vi "DK240 Goto.vi"(4 "StopRef":refnum<vi>, 5 "error in":errorcluster, 6 "Wavelenght":dbl caption="Longueur \nd'onde (nm)" min=0.0 max=16777000.0 step=0.1 format="%#.2f", 7 "MovingRef":refnum<vi>, 8 "Port":refnum<visa-resource-name>="SPECTRO") -> (0 "error out":errorcluster, 2 "Moving":bool caption="Déplacement\nen cours", 3 "Status":u8)   [LabVIEW 2019]
doc: "Goto - Ce Vi commande au réseaux du monochromateur de pivoter à la longueur d'onde désirée, en nm."
uses:
  <vilib>/Utility/error.llb/DialogType.ctl
  <userlib>/GenProg/WritebyWeakRefBool.vi
  <userlib>/GenProg/ReadbyWeakRefBool.vi
panel:
  in  "StopOp":bool
  out "Cancel":u8
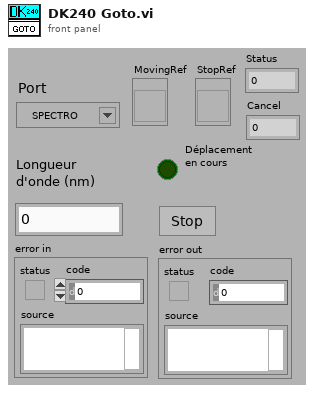
[diagram p1: front panel]
types:
  T1 = enum16{"Commande", "AttendPrêt", "Paramètre", "AttendFin", "Statut", "Fin"}
  T2 = typedef "DialogType.ctl" = u16
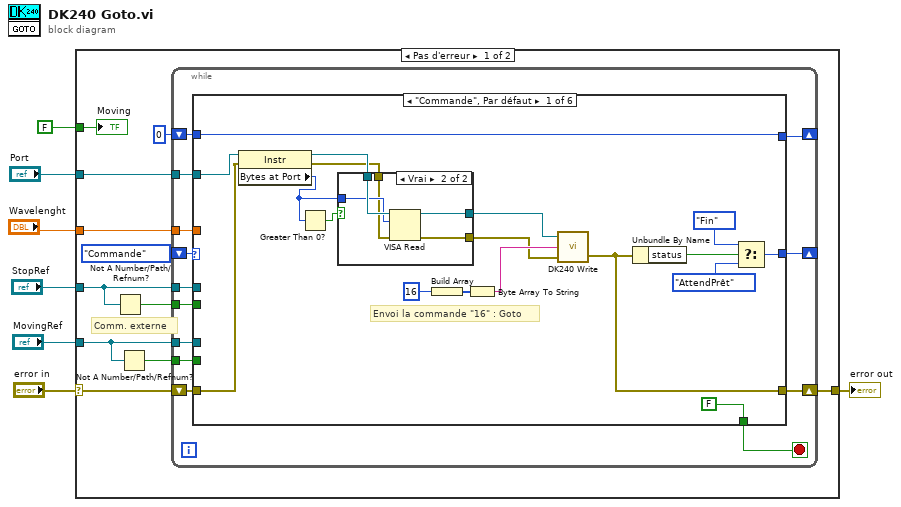
[diagram p0: block diagram]
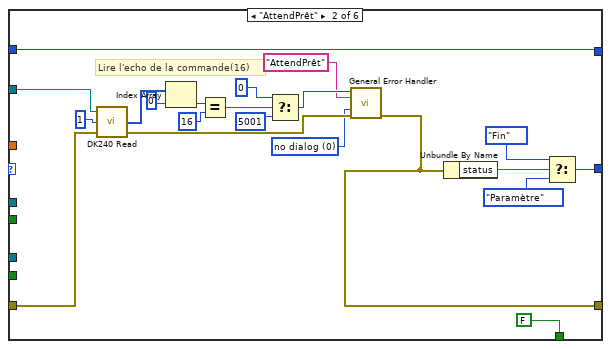
[diagram p3: hidden frame]
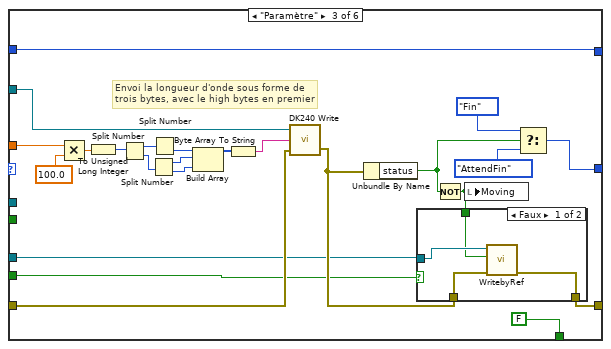
[diagram p4: hidden frame]
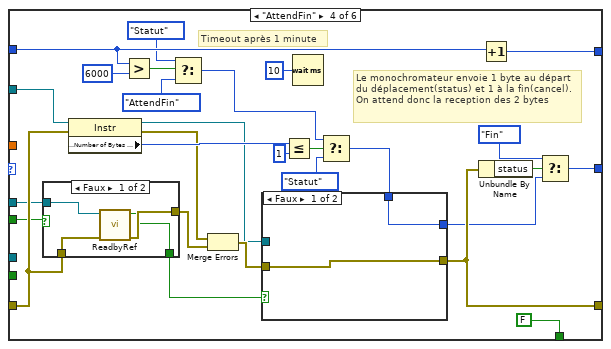
[diagram p6: hidden frame]
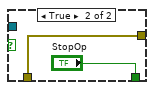
[diagram p7: hidden frame]
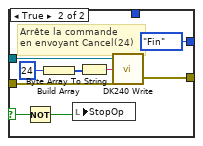
[diagram p8: hidden frame]
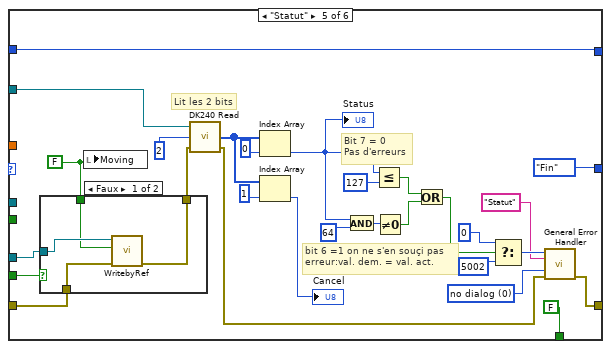
[diagram p9: hidden frame]
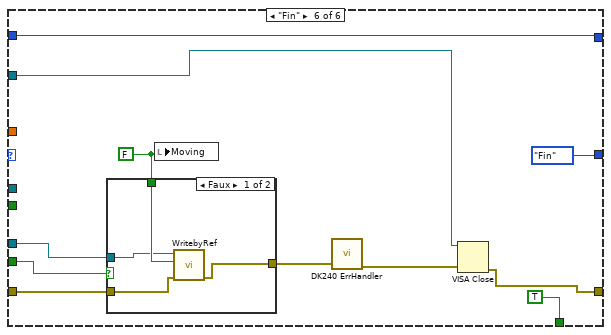
[diagram p11: hidden frame]
diagram:
  n1 = case shown="Pas d'erreur" "error in" {
    selector: "error in" -> [w14 w201]
    tunnel: "Port" -> [w17 _]
    tunnel: "Wavelenght" -> [w16 _]
    tunnel: [w15 w201] -> w6
    tunnel: FALSE ("Moving") -> [w13 _]
    tunnel: "MovingRef" -> [w12 _]
    tunnel: "StopRef" -> [w9 _]
    frame No Error {
      # "Comm. externe"
      n2 = Not A Number/Path/Refnum?(number/path/refnum=w9) -> (NaN/Path/Refnum?=w8:bool)
      n3 = Not A Number/Path/Refnum?(number/path/refnum=w12) -> (NaN/Path/Refnum?=w11:bool)
      n4 = while {
        shift-right: [w27] -> _
        shift-left: T1."Commande" -> [w31]
        tunnel: w17 -> [w30]
        shift-right: [w28] -> w15
        shift-left: w14 -> [w29]
        tunnel: w16 -> [w26]
        tunnel: w12 -> [w24]
        tunnel: w11 -> [w23]
        shift-right: [w22] -> _
        shift-left: 0 -> [w21]
        tunnel: w9 -> [w20]
        tunnel: w8 -> [w19]
        stop <- w25 stop-if-true
        n5 = case shown="\"Commande\", Par défaut" w31 {
          tunnel: w30 -> [w39 w70 w91 w109 w175 w191]
          tunnel: w29 -> [w35 w69 w89 w123 w157 w193]
          tunnel: [w46 w65 w83 w127 w164 w192] -> w28
          tunnel: [w42 w74 w86 w128 T1."Fin" T1."Fin"] -> w27
          tunnel: w26 -> [_ _ w90 _ _ _]
          tunnel: [FALSE FALSE FALSE FALSE FALSE TRUE] -> w25
          tunnel: w24 -> [_ _ w82 _ w154 w190]
          tunnel: w23 -> [_ _ w81 _ w155 w189]
          tunnel: [w40 w57 w78 w118 w152 w187] -> w22
          tunnel: w21 -> [w40 w57 w78 w116 w152 w187]
          tunnel: w20 -> [_ _ _ w110 _ _]
          tunnel: w19 -> [_ _ _ w107 _ _]
          frame "Commande", Default {
            # "Envoi la commande \"16\" : Goto"
            n6 = property class="Instr"(reference=w39, error in=w35) -> (reference out=w37:refnum<visa-resource-name>, error out=w34:errorcluster, "Bytes at Port"=w36:u32)
            n7 = Greater Than 0?(x=w36) -> (x > 0?=w38:bool)
            n8 = case shown="Vrai" w38 {
              tunnel: w37 -> [w50 w56]
              tunnel: w36 -> [_ w55]
              tunnel: w34 -> [w51 w54]
              tunnel: [w51 w53] -> w33
              tunnel: [w50 w52] -> w32
              frame False {
              }
              frame True {
                n9 = VISA Read(VISA resource name=w56, byte count=w55, error in (no error)=w54) -> (VISA resource name out=w52:refnum<visa-resource-name>, error out=w53:errorcluster)  [unwired: 2 out]
              }
            }
            n10 = Build Array(u8 16) -> (w48:u8[])
            n11 = Byte Array To String(unsigned byte array=w48) -> (string=w49:string)
            n12 = call <userlib>:"DK240 Write.vi"("error in"=w33, "String to write"=w49, "Port"=w32) -> ("error out"=w46:errorcluster)  [unwired: 1 in]
            n13 = Unbundle By Name(w46) -> ("status"=w45:bool)
            n14 = Select(t=T1."Fin", s=w45, f=T1."AttendPrêt") -> (s? t:f=w42:T1)
          }
          frame "AttendPrêt" {
            w59 = T2 0 items=["no dialog", "OK message", "continue or stop message", "OK message + warnings", "continue/stop + warnings"] ("type of dialog (OK msg:1)")
            # "Lire l'echo de la commande(16)"
            n15 = call <userlib>:"DK240 Read.vi"("error in"=w69, "Byte count"=u32 1, "Port"=w70) -> ("error out"=w66:errorcluster, "Received Bytes"=w73:u8[])  [unwired: 1 in]
            n16 = Index Array(array=w73, index=0) -> (element=w68:u8)
            n17 = Equal?(x=w68, y=u8 16) -> (x = y?=w64:bool)
            n18 = Select(t=0, s=w64, f=5001 ("t")) -> (s? t:f=w63:i32)
            n19 = call <vilib>:"General Error Handler.vi"("[error code] (0)"=w63, "[error source] (\" \")"="AttendPrêt" ("[error source] (\" \")"), "type of dialog (OK msg:1)"=w59, "error in (no error)"=w66) -> ("error out"=w65:errorcluster)  [unwired: 7 in, 4 out]
            n20 = Unbundle By Name(w65) -> ("status"=w77:bool)
            n21 = Select(t=T1."Fin", s=w77, f=T1."Paramètre") -> (s? t:f=w74:T1)
          }
          frame "Paramètre" {
            # "Envoi la longueur d'onde sous forme de trois bytes, avec le high bytes en premier"
            n22 = Multiply(x=w90, y=100.0) -> (x*y=w99:dbl)
            n23 = To Unsigned Long Integer(number=w99) -> (unsigned 32bit integer=w94:u32)
            n24 = Split Number(x=w94) -> (hi(x)=w93:u16, lo(x)=w92:u16)
            n25 = Split Number(x=w92) -> (hi(x)=w96:u8, lo(x)=w97:u8)
            n26 = Split Number(x=w93) -> (lo(x)=w95:u8)  [unwired: 1 out]
            n27 = Build Array(w95, w96, w97) -> (w100:u8[])
            n28 = Byte Array To String(unsigned byte array=w100) -> (string=w101:string)
            n29 = call <userlib>:"DK240 Write.vi"("error in"=w89, "String to write"=w101, "Port"=w91) -> ("error out"=w84:errorcluster)  [unwired: 1 in]
            n30 = Unbundle By Name(w84) -> ("status"=w79:bool)
            n31 = Not(x=w79) -> (.not. x?=w80:bool)
            n32 = case shown="Faux" w81 {
              tunnel: w82 -> [w105 _]
              tunnel: w84 -> [w103 w106]
              tunnel: [w102 w106] -> w83
              tunnel: w80 -> [w104 _]
              frame False {
                n33 = call-poly <userlib>:"WritebyRef.vi"("error in"=w103, "Valeur"=w104, "Control Ref"=w105) -> ("error out"=w102:errorcluster)  [unwired: 8 in]
              }
              frame True {
              }
            }
            n34 = local write "Moving"(w80) -> ()
            n35 = Select(t=T1."Fin", s=w79, f=T1."AttendFin") -> (s? t:f=w86:T1)
          }
          frame "AttendFin" {
            # "Timeout après 1 minute"
            # "Le monochromateur envoie 1 byte au départ du déplacement(status) et 1 à la fin(cancel). On attend donc la reception des 2 bytes"
            n36 = case shown="Faux" w107 {
              tunnel: w123 -> [w138 w140]
              tunnel: [w135 "StopOp"] -> w120
              tunnel: [w137 w140] -> w119
              tunnel: w110 -> [w136 _]
              frame False {
                n37 = call-poly <userlib>:"ReadbyRef.vi"("error in"=w138, "Control Ref"=w136) -> ("error out"=w137:errorcluster, "Valeur"=w135:bool)  [unwired: 8 in]
              }
              frame True {
              }
            }
            n38 = property class="Instr"(reference=w109, error in=w123) -> (reference out=w108:refnum<visa-resource-name>, error out=w122:errorcluster, "Serial Settings:Number of Bytes at Serial Port"=w134:u32)
            n39 = Greater?(x=w116, y=6000) -> (0:w114:bool)
            n40 = Select(t=T1."Statut", s=w114, f=T1."AttendFin") -> (s? t:f=w111:T1)
            n41 = Merge Errors(w122, w119) -> (w121:errorcluster)
            n42 = Less Or Equal?(x=w134, y=u32 1) -> (x <= y?=w130:bool)
            n43 = Wait (ms)(milliseconds to wait=u32 10) -> ()  [unwired: 1 out]
            n44 = Select(t=w111, s=w130, f=T1."Statut") -> (s? t:f=w125:T1)
            n45 = case shown="Faux" w120 {
              selector: w120 -> [_ w144]
              tunnel: w121 -> [w142 w146]
              tunnel: w108 -> [_ w148]
              tunnel: [w142 w147] -> w127
              tunnel: w125 -> [w141 _]
              tunnel: [w141 T1."Fin"] -> w124
              frame False {
              }
              frame True {
                # "Arrête la commande\nen envoyant Cancel(24)"
                n46 = Not(x=w144) -> (.not. x?=w143:bool)
                n47 = Build Array(u8 24) -> (w150:u8[])
                n48 = local write "StopOp"(w143) -> ()
                n49 = Byte Array To String(unsigned byte array=w150) -> (string=w151:string)
                n50 = call <userlib>:"DK240 Write.vi"("error in"=w146, "String to write"=w151, "Port"=w148) -> ("error out"=w147:errorcluster)  [unwired: 1 in]
              }
            }
            n51 = Unbundle By Name(w127) -> ("status"=w132:bool)
            n52 = Increment(x=w116) -> (x+1=w118:i32)
            n53 = Select(t=T1."Fin", s=w132, f=w124) -> (s? t:f=w128:T1)
          }
          frame "Statut" {
            w169 = T2 0 items=["no dialog", "OK message", "continue or stop message", "OK message + warnings", "continue/stop + warnings"] ("type of dialog (OK msg:1)")
            w153 = FALSE
            # "bit 6 =1 on ne s'en souçi pas \nerreur:val. dem. = val. act."
            # "Bit 7 = 0\nPas d'erreurs"
            # "Lit les 2 bits"
            n54 = case shown="Faux" w155 {
              tunnel: w157 -> [w181 w184]
              tunnel: [w180 w184] -> w156
              tunnel: w154 -> [w183 _]
              tunnel: w153 -> [w182 _]
              frame False {
                n55 = call-poly <userlib>:"WritebyRef.vi"("error in"=w181, "Valeur"=w182, "Control Ref"=w183) -> ("error out"=w180:errorcluster)  [unwired: 8 in]
              }
              frame True {
              }
            }
            n56 = local write "Moving"(w153) -> ()
            n57 = call <userlib>:"DK240 Read.vi"("error in"=w156, "Byte count"=u32 2, "Port"=w175) -> ("error out"=w168:errorcluster, "Received Bytes"=w179:u8[])  [unwired: 1 in]
            n58 = Index Array(array=w179, index=0) -> (element=w160:u8)
            "Status" <- w160
            n59 = Index Array(array=w179, index=1) -> (element=→"Cancel":u8)
            n60 = And(x=w160, y=u8 64) -> (x .and. y?=w166:u8)
            n61 = Less Or Equal?(x=w160, y=u8 127) -> (x <= y?=w163:bool)
            n62 = Not Equal To 0?(x=w166) -> (x != 0?=w162:bool)
            n63 = Or(x=w163, y=w162) -> (x .or. y?=w161:bool)
            n64 = Select(t=0, s=w161, f=5002 ("t")) -> (s? t:f=w173:i32)
            n65 = call <vilib>:"General Error Handler.vi"("[error code] (0)"=w173, "[error source] (\" \")"="Statut" ("[error source] (\" \")"), "type of dialog (OK msg:1)"=w169, "error in (no error)"=w168) -> ("error out"=w164:errorcluster)  [unwired: 7 in, 4 out]
          }
          frame "Fin" {
            w188 = FALSE
            n66 = case shown="Faux" w189 {
              tunnel: w190 -> [w198 _]
              tunnel: w193 -> [w197 w200]
              tunnel: [w196 w200] -> w186
              tunnel: w188 -> [w199 _]
              frame False {
                n67 = call-poly <userlib>:"WritebyRef.vi"("error in"=w197, "Valeur"=w199, "Control Ref"=w198) -> ("error out"=w196:errorcluster)  [unwired: 8 in]
              }
              frame True {
              }
            }
            n68 = local write "Moving"(w188) -> ()
            n69 = call <userlib>:"DK240 ErrHandler.vi"("error in"=w186) -> ("error out"=w185:errorcluster)  [unwired: 7 in]
            n70 = VISA Close(VISA resource name=w191, error in (no error)=w185) -> (error out=w192:errorcluster)
          }
        }
      }
      "Moving" <- w13
    }
    frame Error {
    }
  }
  "error out" <- w6
